vi "astrometry.vi"(11 "Astrometry":T2) -> ()   [LabVIEW 2010]
uses:
  <vilib>/Analysis/Matrix/Datatypes/RealMatrix.ctl
  <vilib>/Analysis/Matrix/Numeric/Conversions/Array To Matrix - RA2.vi
  <vilib>/Analysis/baseanly.llb/Real Determinant.vi
  <vilib>/Analysis/Matrix/NI_Matrix.lvlib
  <vilib>/Analysis/NI_AALBase.lvlib
panel:
  out "Inverse Matrix":T1
  out "scale":dbl
  out "cd_det":dbl format="%.2e"
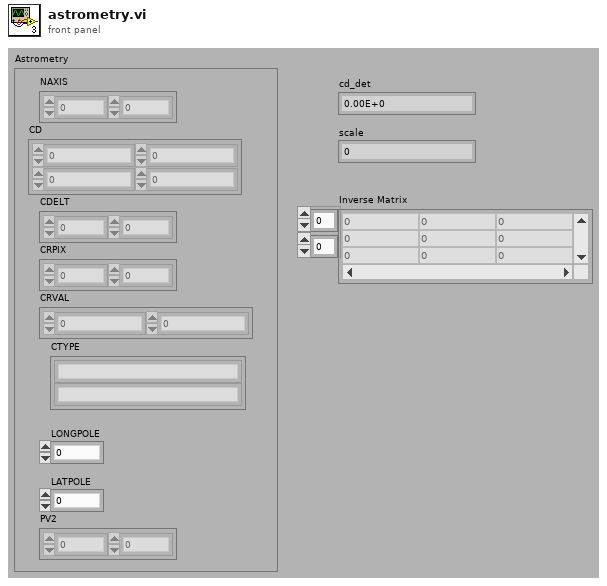
[diagram p1: front panel]
types:
  T1 = typedef "NI_Matrix.lvlib/RealMatrix.ctl" = dbl[][]
  T2 = cluster{"NAXIS":dbl[], "CD":dbl[][], "CDELT":dbl[], "CRPIX":dbl[], "CTYPE":string[], "CRVAL":dbl[], "LONGPOLE":dbl, "LATPOLE":dbl, "PV2":dbl[]}
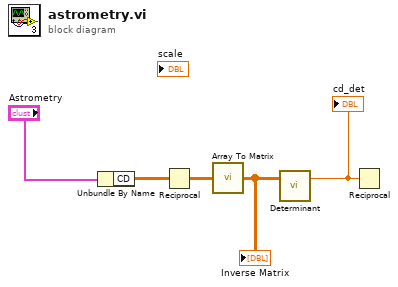
[diagram p0: block diagram]
diagram:
  n1 = Unbundle By Name("Astrometry") -> ("CD"=w3:dbl[][])
  n2 = Reciprocal(x=w3) -> (1/x=w2:dbl[][])
  n3 = call-poly <vilib>:"Array To Matrix.vi"("Real 2D Array"=w2) -> ("Real Matrix"=w4:T1)
  "Inverse Matrix" <- w4
  n4 = call-poly <vilib>:"Determinant.vi"("Input Matrix"=w4) -> ("determinant"=w1:dbl)  [unwired: 1 in, 1 out]
  "cd_det" <- w1
  n5 = Reciprocal(x=w1) -> ()  [unwired: 1 out]
